vi "Configure Analog References.vi"(5 "Watts Reference Impedance (8 ohms)":dbl=8.0, 6 "Decibel Reference Impedance (600 ohms)":dbl=600.0, 7 "Analog Frequency (10 mHz)":dbl=10.0, 8 "error in (no error)":errorcluster, 9 "Decibel Reference B (1 dBrB)":dbl=1.0, 10 "Decibel Reference A (1 dBrA)":dbl=1.0, 11 "VISA resource name":refnum<visa-resource-name>) -> (0 "error out":errorcluster, 3 "VISA resource name out":refnum<visa-resource-name>)   [LabVIEW 2014, in "Stanford Research SR1.lvlib"]
doc: "Configures the Analog References for the Analyzer."
uses:
  Stanford Research SR1.lvlib
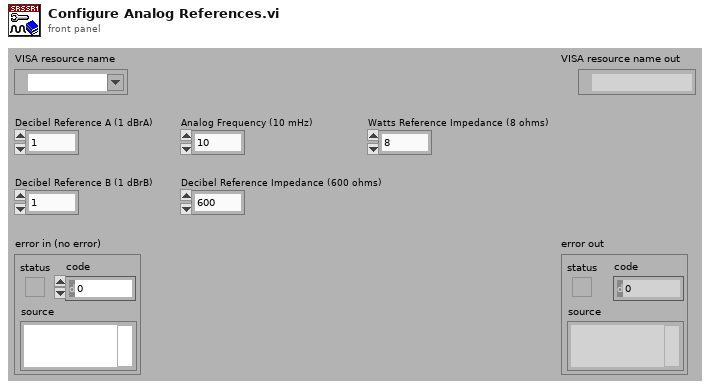
[diagram p1: front panel]
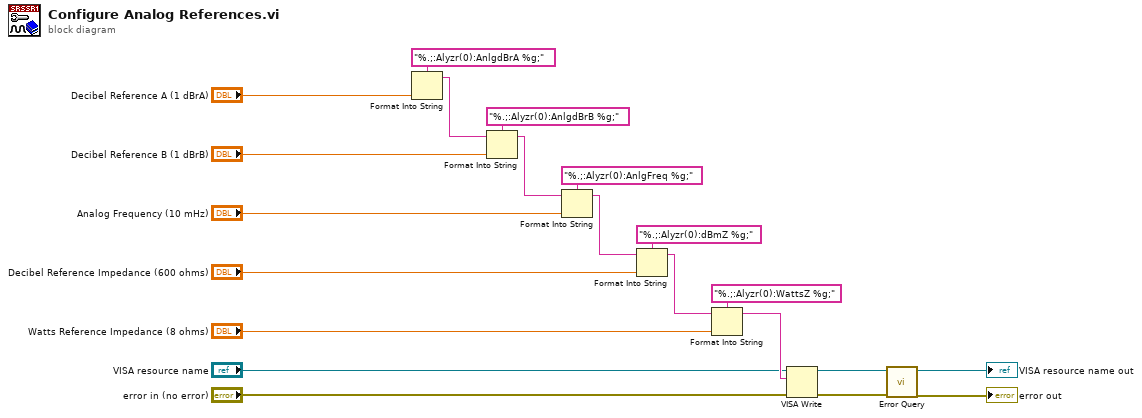
[diagram p0: block diagram]
diagram:
  n1 = Format Into String(format string="%.;:Alyzr(0):AnlgdBrA %g;", "Decibel Reference A (1 dBrA)") -> (resulting string=w19:string)  [unwired: 2 in, 1 out]
  n2 = Format Into String(format string="%.;:Alyzr(0):AnlgdBrB %g;", initial string=w19, "Decibel Reference B (1 dBrB)") -> (resulting string=w16:string)  [unwired: 1 in, 1 out]
  n3 = Format Into String(format string="%.;:Alyzr(0):AnlgFreq %g;", initial string=w16, "Analog Frequency (10 mHz)") -> (resulting string=w13:string)  [unwired: 1 in, 1 out]
  n4 = Format Into String(format string="%.;:Alyzr(0):dBmZ %g;", initial string=w13, "Decibel Reference Impedance (600 ohms)") -> (resulting string=w10:string)  [unwired: 1 in, 1 out]
  n5 = Format Into String(format string="%.;:Alyzr(0):WattsZ %g;", initial string=w10, "Watts Reference Impedance (8 ohms)") -> (resulting string=w7:string)  [unwired: 1 in, 1 out]
  n6 = VISA Write(VISA resource name="VISA resource name", write buffer=w7, error in (no error)="error in (no error)") -> (VISA resource name out=w4:refnum<visa-resource-name>, error out=w3:errorcluster)  [unwired: 1 out]
  n7 = call "Error Query.vi"("error in (no error)"=w3, "VISA resource name"=w4) -> ("error out"=→"error out":errorcluster, "VISA resource name out"=→"VISA resource name out":refnum<visa-resource-name>)  [unwired: 6 in, 2 out]
